vi "Update States.vi"(8 "error in (no error)":errorcluster, 10 "Initialize?":bool, 11 "Engine Data in":T1) -> (0 "error out":errorcluster, 3 "Engine Data out":T1)   [LabVIEW 2020, in "Routing and Faulting Engine.lvlib"]
uses:
  Routing and Faulting Engine.lvlib
  Engine Data.ctl
  Includes/CDMessaging.lvlibp/Producer/Abstract Producer/Abstract Producer.lvclass
  Shared/Compiled.Settings.ctl
  Shared/Communication Configuration.ctl
  Shared/Routing and Faulting Configuration.ctl
  Shared/Routing Channel Configuration.ctl
  Shared/Value-Connections Map.ctl
  Shared/Alias Mapping.ctl
  Shared/Alias Endpoint.ctl
  Shared/Compiled Connection.ctl
  Shared/FIFO Indices.ctl
  Device Inputs.ctl
  Device Outputs.ctl
  Shared/Routing and Faulting Shared.lvlib
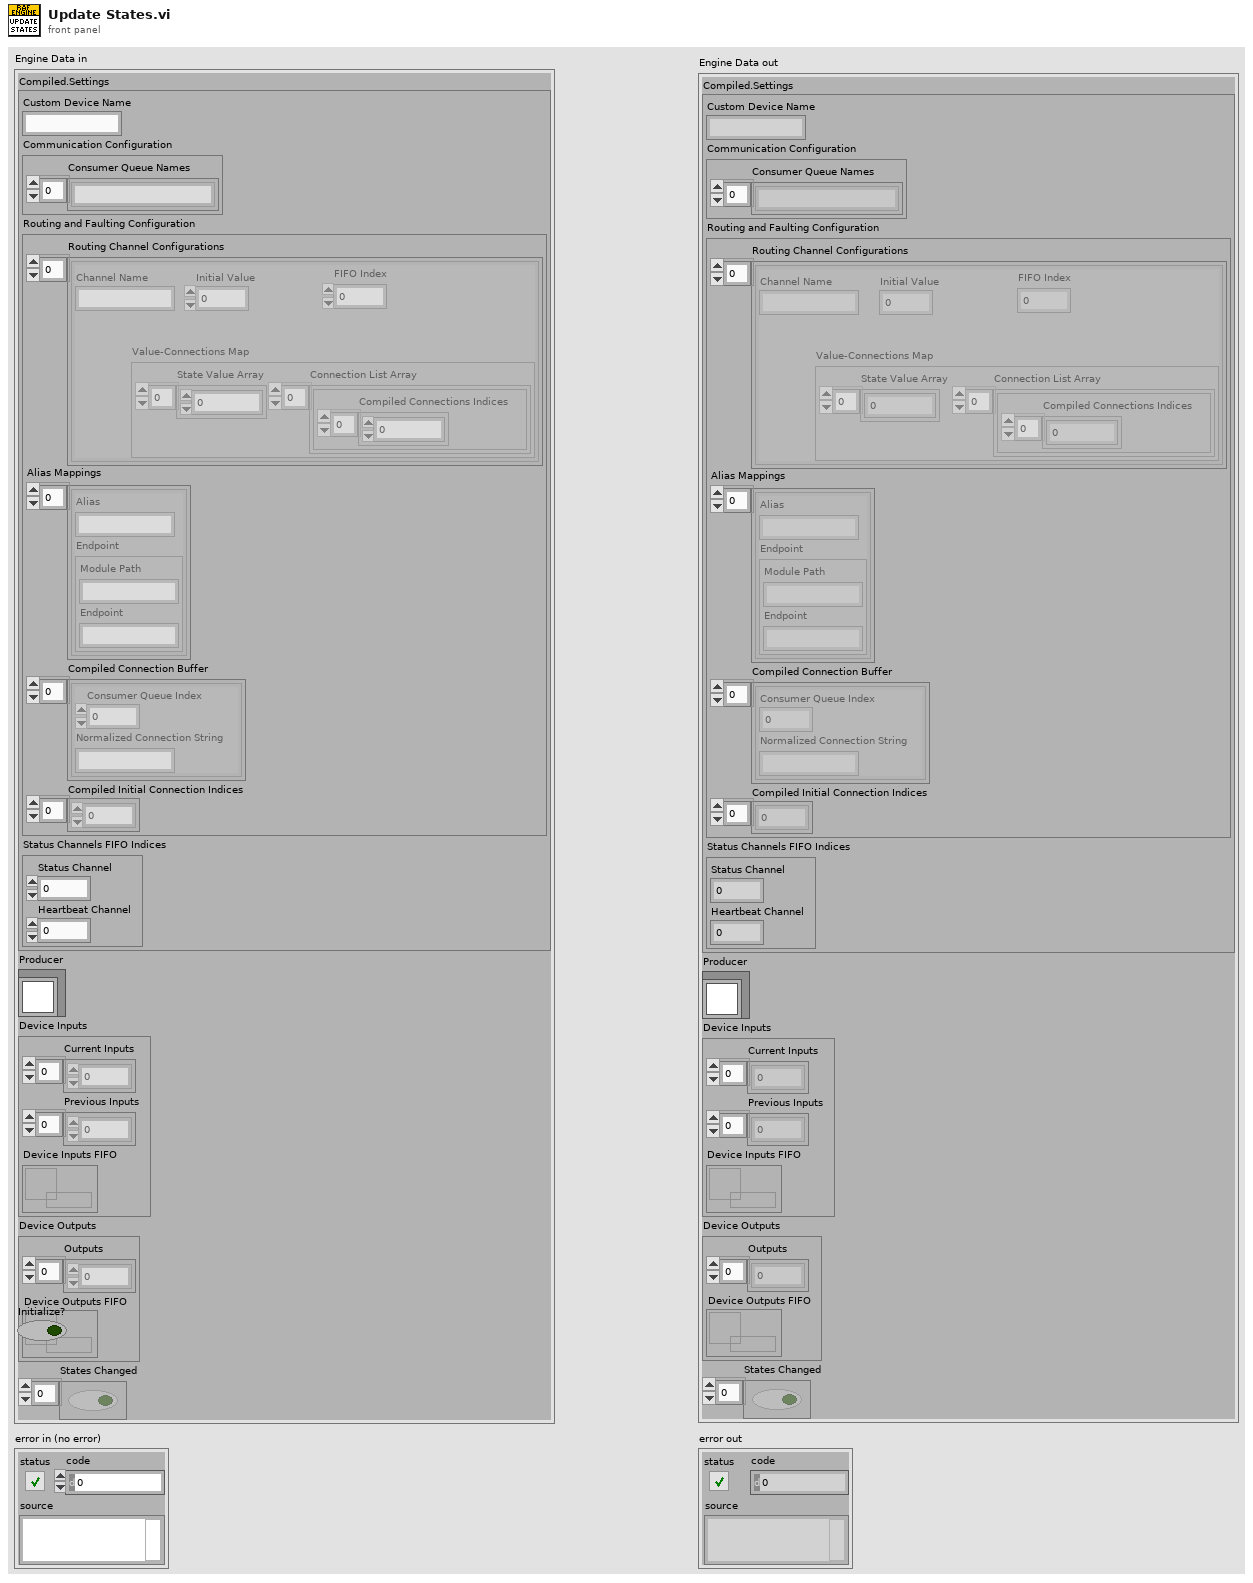
[diagram p1: front panel]
types:
  T1 = typedef "Routing and Faulting Engine.lvlib/Engine Data.ctl" = cluster{"Compiled.Settings":T2, "Producer":refnum<class "Abstract Producer.lvclass">, "Device Inputs":T11, "Device Outputs":T12, "States Changed":bool[]}
  T2 = typedef "Routing and Faulting Shared.lvlib/Compiled.Settings.ctl" = cluster{"Custom Device Name":string, "Communication Configuration":T3, "Routing and Faulting Configuration":T4, "Status Channels FIFO Indices":T10}
  T3 = typedef "Routing and Faulting Shared.lvlib/Communication Configuration.ctl" = cluster{"Consumer Queue Names":string[]}
  T4 = typedef "Routing and Faulting Shared.lvlib/Routing and Faulting Configuration.ctl" = cluster{"Routing Channel Configurations":T5[], "Alias Mappings":T7[], "Compiled Connection Buffer":T9[], "Compiled Initial Connection Indices":i32[]}
  T5 = typedef "Routing and Faulting Shared.lvlib/Routing Channel Configuration.ctl" = cluster{"Channel Name":string, "Initial Value":dbl, "FIFO Index":i32, "Value-Connections Map":T6}
  T6 = typedef "Routing and Faulting Shared.lvlib/Value-Connections Map.ctl" = cluster{"State Value Array":i32[], "Connection List Array":cluster{"Compiled Connections Indices":i32[]}[]}
  T7 = typedef "Routing and Faulting Shared.lvlib/Alias Mapping.ctl" = cluster{"Alias":string, "Endpoint":T8}
  T8 = typedef "Routing and Faulting Shared.lvlib/Alias Endpoint.ctl" = cluster{"Module Path":string, "Endpoint":string}
  T9 = typedef "Routing and Faulting Shared.lvlib/Compiled Connection.ctl" = cluster{"Consumer Queue Index":i32, "Normalized Connection String":string}
  T10 = typedef "Routing and Faulting Shared.lvlib/FIFO Indices.ctl" = cluster{"Status Channel":i32, "Heartbeat Channel":i32}
  T11 = typedef "Routing and Faulting Engine.lvlib/Device Inputs.ctl" = cluster{"Current Inputs":dbl[], "Previous Inputs":dbl[], "Device Inputs FIFO":refnum<k33>}
  T12 = typedef "Routing and Faulting Engine.lvlib/Device Outputs.ctl" = cluster{"Outputs":dbl[], "Device Outputs FIFO":refnum<k33>}
  T13 = typedef "Routing and Faulting Engine.lvlib/Producer Message.ctl" = cluster{"Consumer":string, "Message":refnum<class "Abstract Message.lvclass">}
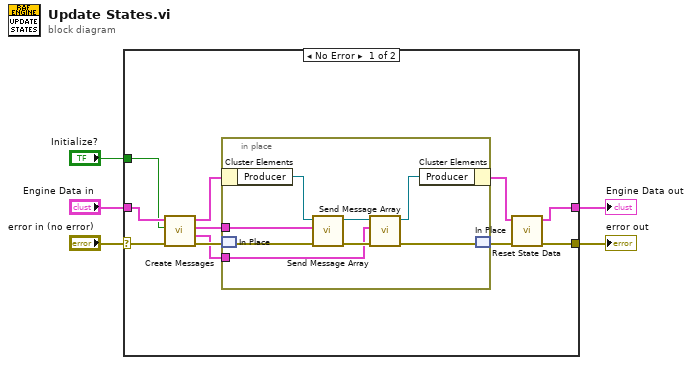
[diagram p0: block diagram]
diagram:
  n1 = case shown="No Error" "error in (no error)" {
    selector: "error in (no error)" -> [w14 w26]
    tunnel: "Engine Data in" -> [w13 w25]
    tunnel: [w16 w26] -> w3
    tunnel: [w15 w25] -> w2
    tunnel: "Initialize?" -> [w6 _]
    frame No Error {
      n2 = call "Create Messages.vi"("error in (no error)"=w14, "Initialize?"=w6, "Engine Data in"=w13) -> ("error out"=w12:errorcluster, "Connect Messages"=w9:T13[], "Disconnect Messages"=w10:T13[], "Engine Data out"=w8:T1)  [unwired: 5 in]
      n3 = in-place {
        in-place-border: w10 -> [w18]
        in-place-border: w9 -> [w17]
        n4 = in-place-cluster #1(w8) -> ("Producer"=w23:refnum<class "Abstract Producer.lvclass">)
        n5 = in-place-match #2(w12) -> (w24:errorcluster)
        n6 = call "Send Message Array.vi"("error in (no error)"=w24, "Message Array"=w18, "Producer in"=w23) -> ("error out"=w22:errorcluster, "Producer out"=w21:refnum<class "Abstract Producer.lvclass">)  [unwired: 7 in]
        n7 = call "Send Message Array.vi"("error in (no error)"=w22, "Message Array"=w17, "Producer in"=w21) -> ("error out"=w20:errorcluster, "Producer out"=w19:refnum<class "Abstract Producer.lvclass">)  [unwired: 7 in]
        n8 = in-place-cluster #1("Producer"=w19) -> (w7:T1)
        n9 = in-place-match #2(w20) -> (w11:errorcluster)
      }
      n10 = call "Reset State Data.vi"("error in (no error)"=w11, "Engine Data in"=w7) -> ("error out"=w16:errorcluster, "Engine Data out"=w15:T1)  [unwired: 8 in]
    }
    frame Error {
    }
  }
  "Engine Data out" <- w2
  "error out" <- w3
